vi "getRecordsFrombuffer.vi"(0 "data in":string) -> (4 "foundPack":u8[][](array[numeric]), 6 "index of Sync":i32[](array[numeric]), 8 "remaining data":string, 10 "remaining data?":bool, 15 "Found":i32)   [LabVIEW 2023]
uses:
  c702e427-e749-45d1-876f-7929ce429696.vi
  <vilib>/Comparison/Equal/Equal Functor/Equal Functor.lvclass
panel:
  out "unsigned 16bit integer":u16
  out "size(s)":i32
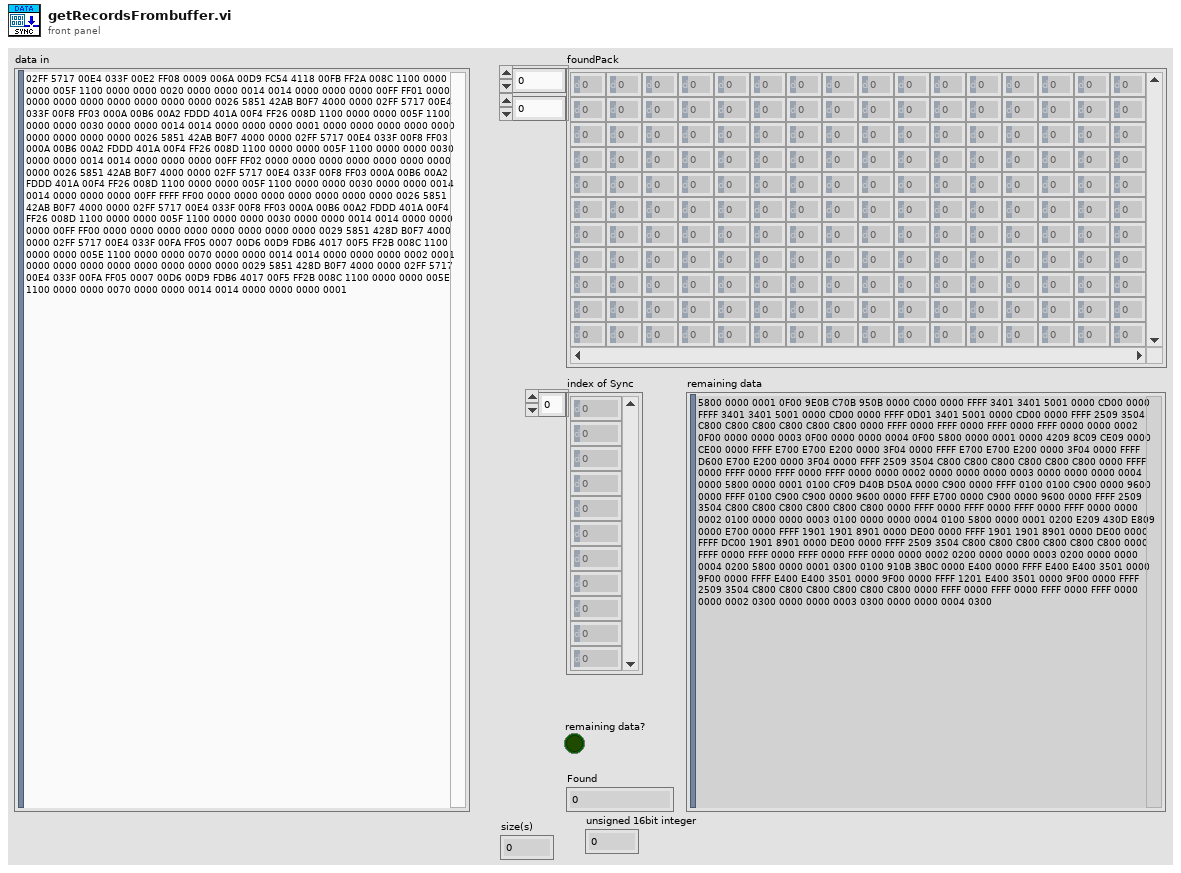
[diagram p1: front panel]
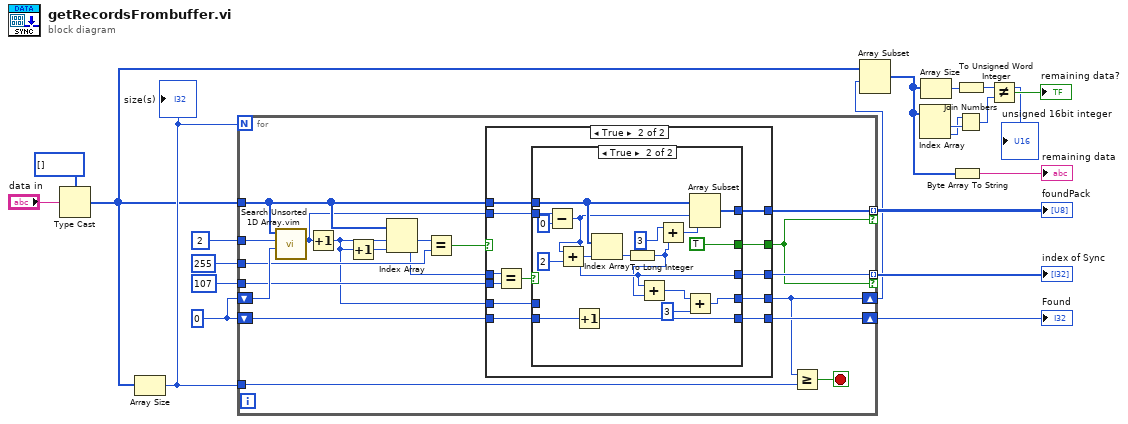
[diagram p0: block diagram]
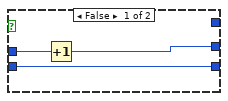
[diagram p3: hidden frame]
diagram:
  w15 = 0 ("start index (0)")
  n1 = Type Cast(type=u8[] [], x="data in") -> (*(type *) &x=w3:u8[])
  n2 = Array Size(array=w3) -> (size(s)=w13:i32)
  "size(s)" <- w13
  n3 = for {
    N: w13 -> [_]
    tunnel: w3 -> [w33]
    tunnel: u8 2 -> [w39]
    shift-right: [w30] -> w2
    shift-left: w15 -> [w37]
    tunnel: u8 255 -> [w36]
    tunnel: u8 107 -> [w34]
    tunnel: [w23] -> w11 mode=indexing if=w21
    shift-right: [w32] -> w14
    shift-left: w15 -> [w22]
    tunnel: [w31] -> w12 mode=indexing if=w21
    tunnel: w13 -> [w27]
    stop <- w24 stop-if-true
    n4 = call "Search Unsorted 1D Array.vim"("start index (0)"=w37, "element"=w39, "unsorted 1D array"=w33) -> ("index of element"=w26:i32)  [unwired: 8 in]
    n5 = Increment(x=w26) -> (x+1=w29:i32)
    n6 = Increment(x=w29) -> (x+1=w28:i32)
    n7 = Index Array(array=w33, index #1=w29, index #2=w28) -> (element #1=w38:u8, element #2=w35:u8)
    n8 = Equal?(x=w38, y=w36) -> (x = y?=w25:bool)
    n9 = case shown="True" w25 {
      tunnel: w35 -> [_ w53]
      tunnel: w34 -> [_ w52]
      tunnel: [w40 w49] -> w30
      tunnel: w29 -> [w40 w50]
      tunnel: w33 -> [_ w48]
      tunnel: w26 -> [_ w47]
      tunnel: [_ w46] -> w23
      tunnel: [_ w45] -> w21
      tunnel: w22 -> [w41 w44]
      tunnel: [w41 w43] -> w32
      tunnel: [_ w42] -> w31
      frame False {
      }
      frame True {
        n10 = Equal?(x=w53, y=w52) -> (x = y?=w51:bool)
        n11 = case shown="True" w51 {
          tunnel: w50 -> [w55 _]
          tunnel: [w54 w60] -> w49
          tunnel: w48 -> [_ w70]
          tunnel: w47 -> [_ w73]
          tunnel: [_ w67] -> w46
          tunnel: [_ TRUE] -> w45
          tunnel: w44 -> [w56 w69]
          tunnel: [w56 w68] -> w43
          tunnel: [_ w63] -> w42
          frame False {
            n12 = Increment(x=w55) -> (x+1=w54:i32)
          }
          frame True {
            n13 = Subtract(x=w73, y=0) -> (x-y=w63:i32)
            n14 = Add(x=w63, y=2) -> (x+y=w65:i32)
            n15 = Increment(x=w69) -> (x+1=w68:i32)
            n16 = Index Array(array=w70, index=w65) -> (element=w64:u8)
            n17 = To Long Integer(number=w64) -> (32bit integer=w59:i32)
            n18 = Add(x=w63, y=w59) -> (x+y=w62:i32)
            n19 = Add(x=3 ("y"), y=w59) -> (x+y=w57:i32)
            n20 = Add(x=w62, y=3) -> (x+y=w60:i32)
            n21 = Array Subset(array=w70, index=w63, length=w57) -> (w67:u8[])
          }
        }
      }
    }
    n22 = Greater Or Equal?(x=w30, y=w27) -> (x >= y?=w24:bool)
  }
  "foundPack" <- w11
  "Found" <- w14
  "index of Sync" <- w12
  n23 = Array Subset(array=w3, index=w2) -> (w1:u8[])  [unwired: 1 in]
  n24 = Index Array(array=w1) -> (element #1=w8:u8, element #2=w7:u8)  [unwired: 2 in]
  n25 = Array Size(array=w1) -> (size(s)=w6:i32)
  n26 = Byte Array To String(unsigned byte array=w1) -> (string=→"remaining data":string)
  n27 = To Unsigned Word Integer(number=w6) -> (unsigned 16bit integer=w5:u16)
  "unsigned 16bit integer" <- w5
  n28 = Join Numbers(hi=w7, lo=w8) -> ((hi.lo)=w9:u16)
  n29 = Not Equal?(x=w5, y=w9) -> (x != y?=→"remaining data?":bool)
